vi "Read Msg Self.vi"(11 "Actor in":refnum<class "Actor.lvclass">) -> (2 "Msg Self":refnum<class "Msg Self.lvclass">)   [LabVIEW 2020, in "jettl.lvlib" / "Actor.lvclass"]
uses:
  Actor.lvclass
  Msg Self/Msg Self.lvclass
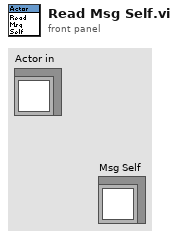
[diagram p1: front panel]
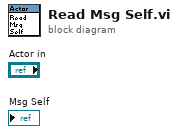
[diagram p0: block diagram]
diagram:
